vi "Input Personal Detail.vi"(6 "Error In":errorcluster) -> (0 "Error Out":errorcluster, 1 "Terminate":bool, 2 "Test Info":T2, 3 "Simulated Data?":bool)   [LabVIEW 2017]
uses:
  <vilib>/Utility/miscctls.llb/LVRectTypeDef.ctl
panel:
  in  "Path":path=path "C:/Labtech"
  in  "Comments":string
  in  "Panel Bounds":T1={"Left"=0, "Top"=0, "Right"=500, "Bottom"=500}
  in  "Boolean":bool
  out "Instructions":bool
  in  "Date":string
  in  "stop 2":bool
  in  "Test Name":string
  in  "Test ID":string
  in  "Customer":string
  in  "SPN":string
  in  "Operator Name":string
  # "Test Information"
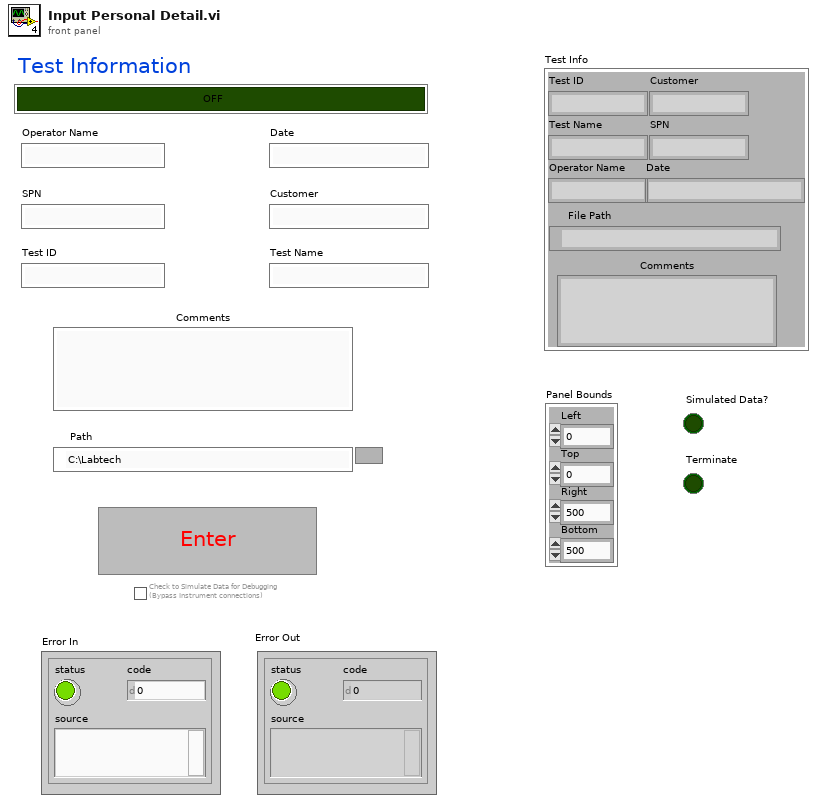
[diagram p1: front panel]
types:
  T1 = typedef "LVRectTypeDef.ctl" = cluster{"Left":i16, "Top":i16, "Right":i16, "Bottom":i16}
  T2 = cluster{"Test ID":string, "Test Name":string, "Customer":string, "SPN":string, "Operator Name":string, "Date":string, "File Path":path, "Comments":string}
  T3 = enum32{"existing file", "new file", "new or existing file", "existing dir", "new dir", "new or existing dir", "existing file (use LLBs)", "new file (use LLBs)", "new or existing file (use LLBs)", "new or existing file or directory (use LLBs)", "existing dir (use LLBs)", "new dir (use LLBs)", "new or existing dir (use LLBs)", "existing file or dir", "new file or dir", "new or existing file or dir", "existing file or dir (use LLBs)", "new file or dir (use LLBs)"}
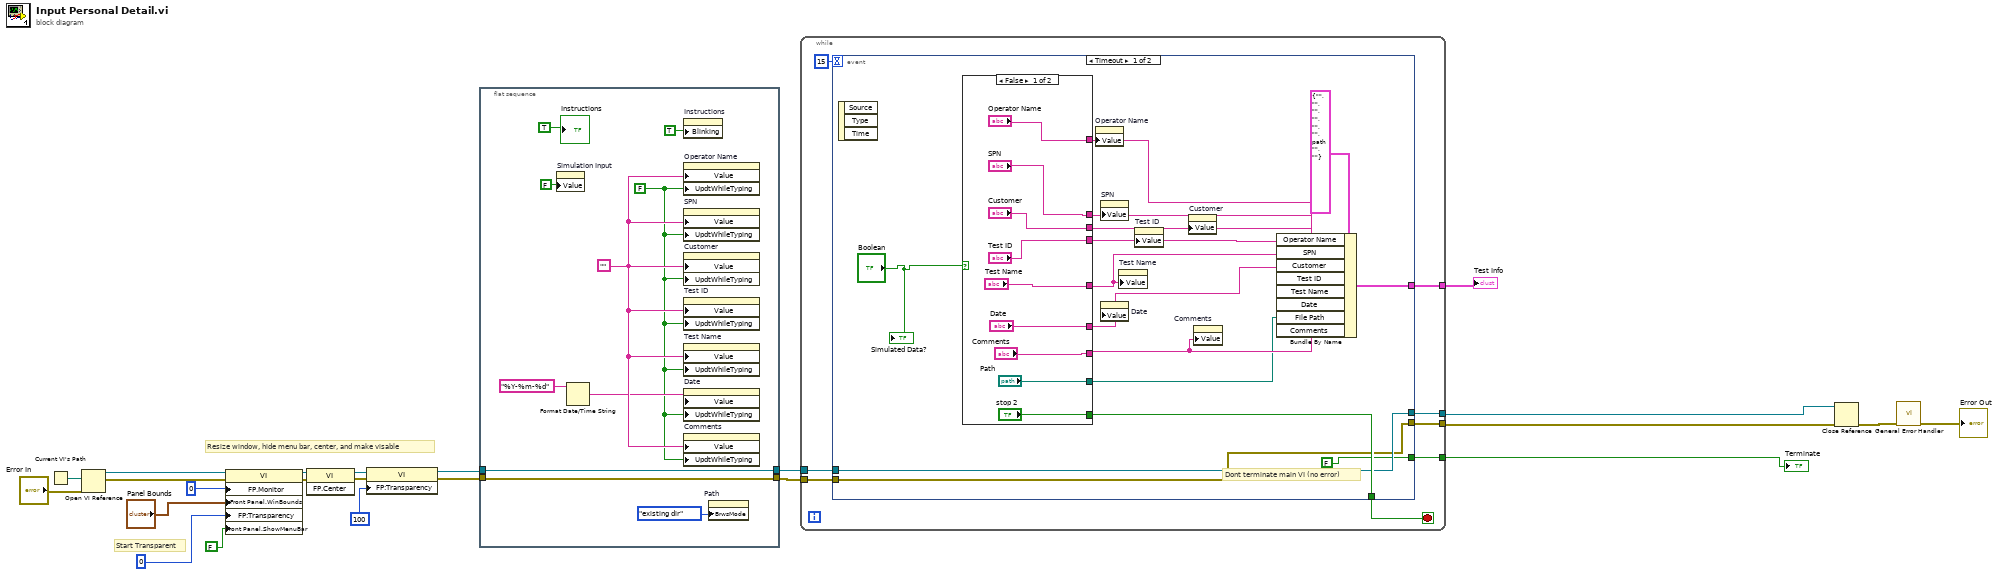
[diagram p0: block diagram]
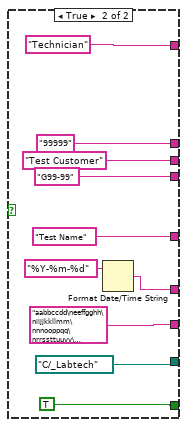
[diagram p2: hidden frame]
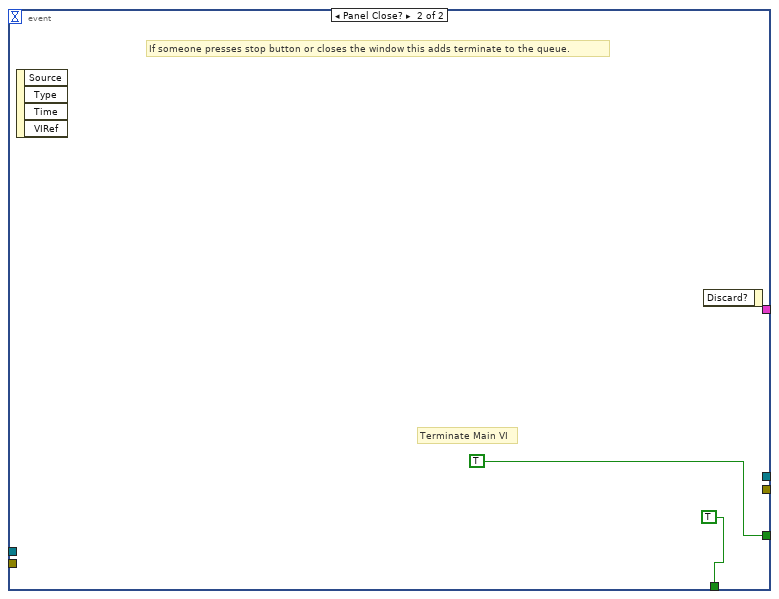
[diagram p3: hidden frame]
diagram:
  # "Resize window, hide menu bar, center, and make visable"
  # "Start Transparent"
  n1 = Current VI's Path() -> (path=w22:path)
  n2 = Open VI Reference(vi path=w22, error in (no error)="Error In") -> (vi reference=w21:refnum<vi>, error out=w20:errorcluster)  [unwired: 4 in]
  n3 = property class="VI"(reference=w21, error in=w20, "FP.Monitor"=0, "Front Panel.WinBounds"="Panel Bounds", "FP:Transparency"=0, "Front Panel.ShowMenuBar"=FALSE) -> (reference out=w17:refnum<vi>, error out=w16:errorcluster)
  n4 = invoke class="VI" method="FP.Center"(reference=w17, error in=w16) -> (reference out=w15:refnum<vi>, error out=w14:errorcluster)  [unwired: 1 in, 1 out]
  n5 = property class="VI"(reference=w15, error in=w14, "FP:Transparency"=100) -> (reference out=w2:refnum<vi>, error out=w3:errorcluster)
  n6 = flat-sequence {
    tunnel: w3 -> [w33]
    tunnel: [w33] -> w23
    tunnel: [w29] -> w8
    tunnel: w2 -> [w29]
    frame #0 {
      w25 = FALSE ("Update While Typing?")
      w28 = ""
      n7 = property on="Simulation Input" class="Bool (strict)"("Value"=FALSE) -> ()  [unwired: 2 in, 2 out]
      n8 = Format Date/Time String(time format string (%c)="%Y-%m-%d") -> (date/time string=w27:string)  [unwired: 2 in]
      n9 = property on="Instructions" class="Bool (strict)"("Blinking"=TRUE) -> ()  [unwired: 2 in, 2 out]
      n10 = property on="Operator Name" class="Str"("Value"=w28, "UpdtWhileTyping"=w25) -> ()  [unwired: 2 in, 2 out]
      n11 = property on="SPN" class="Str"("Value"=w28, "UpdtWhileTyping"=w25) -> ()  [unwired: 2 in, 2 out]
      n12 = property on="Customer" class="Str"("Value"=w28, "UpdtWhileTyping"=w25) -> ()  [unwired: 2 in, 2 out]
      n13 = property on="Test ID" class="Str"("Value"=w28, "UpdtWhileTyping"=w25) -> ()  [unwired: 2 in, 2 out]
      n14 = property on="Test Name" class="Str"("Value"=w28, "UpdtWhileTyping"=w25) -> ()  [unwired: 2 in, 2 out]
      n15 = property on="Date" class="Str"("Value"=w27, "UpdtWhileTyping"=w25) -> ()  [unwired: 2 in, 2 out]
      n16 = property on="Comments" class="Str"("Value"=w28, "UpdtWhileTyping"=w25) -> ()  [unwired: 2 in, 2 out]
      n17 = property on="Path" class="Path"("BrwsMode"=T3."existing dir" ("Browse Options:Selection Mode")) -> ()  [unwired: 2 in, 2 out]
      "Instructions" <- TRUE
    }
  }
  n18 = while {
    tunnel: w23 -> [w40]
    tunnel: [w39] -> w6
    tunnel: w8 -> [w37]
    tunnel: [w38] -> w4
    tunnel: [w36] -> w7
    tunnel: [w34] -> w1
    stop <- w41 stop-if-true
    n19 = event shown="[0] Timeout" {
      selector: _ -> [_ _]
      dyn-events: _ -> [_ _]
      timeout: 15 -> [_ _]
      tunnel: [w50 TRUE] -> w41
      tunnel: w40 -> [w47 _]
      tunnel: [w47 _] -> w39
      tunnel: w37 -> [w48 _]
      tunnel: [w48 _] -> w38
      tunnel: [FALSE TRUE] -> w36
      tunnel: [w42 _] -> w34
      event Timeout {
        # "Dont terminate main VI (no error)"
        n20 = event-data() -> ()  [unwired: 1 in, 3 out]
        n21 = case shown="False" "Boolean" {
          tunnel: ["Operator Name" "Technician"] -> w56
          tunnel: ["SPN" "99999"] -> w51
          tunnel: ["Customer" "Test Customer"] -> w52
          tunnel: ["Test ID" "G99-99"] -> w53
          tunnel: ["Test Name" "Test Name"] -> w54
          tunnel: ["Date" w66] -> w55
          tunnel: ["stop 2" TRUE] -> w50
          tunnel: ["Comments" "aabbccdd\neeffgghh\niijjkkllmm\nnnooppqq\nrrssttuuvv\nwwxxyyzz"] -> w44
          tunnel: ["Path" path "C:/_Labtech"] -> w43
          frame False {
          }
          frame True {
            n22 = Format Date/Time String(time format string (%c)="%Y-%m-%d") -> (date/time string=w66:string)  [unwired: 2 in]
          }
        }
        n23 = property on="Operator Name" class="Str"("Value"=w56) -> ()  [unwired: 2 in, 2 out]
        n24 = property on="SPN" class="Str"("Value"=w51) -> ()  [unwired: 2 in, 2 out]
        n25 = property on="Date" class="Str"("Value"=w55) -> ()  [unwired: 2 in, 2 out]
        n26 = property on="Test Name" class="Str"("Value"=w54) -> ()  [unwired: 2 in, 2 out]
        n27 = property on="Test ID" class="Str"("Value"=w53) -> ()  [unwired: 2 in, 2 out]
        n28 = property on="Customer" class="Str"("Value"=w52) -> ()  [unwired: 2 in, 2 out]
        n29 = property on="Comments" class="Str"("Value"=w44) -> ()  [unwired: 2 in, 2 out]
        n30 = Bundle By Name(cluster=T2 {"Test ID"="", "Test Name"="", "Customer"="", "SPN"="", "Operator Name"="", "Date"="", "File Path"=path "", "Comments"=""} ("output cluster 2"), "Operator Name"=w56, "SPN"=w51, "Customer"=w52, "Test ID"=w53, "Test Name"=w54, "Date"=w55, "File Path"=w43, "Comments"=w44) -> (w42:T2)
        "Simulated Data?" <- "Boolean"
      }
      event Panel Close? {
        # "Terminate Main VI"
        # "If someone presses stop button or closes the window this adds terminate to the queue."
        n31 = event-data() -> ()  [unwired: 1 in, 4 out]
        n32 = event-data() -> ()  [unwired: 2 in, 1 out]
      }
    }
  }
  "Terminate" <- w7
  "Test Info" <- w1
  n33 = Close Reference(reference=w4, error in (no error)=w6) -> (error out=w5:errorcluster)
  n34 = call <vilib>:"General Error Handler.vi"("error in (no error)"=w5) -> ("error out"=→"Error Out":errorcluster)  [unwired: 10 in, 4 out]
